vi "Fix_multi_header_bug.vi"(1 "Raw data File to Read":path) -> (0 "Raw data File to Read Out":path)   [LabVIEW 2018]
uses:
  Globals/Meas_global.vi
  Globals/Constants_global.vi
panel:
  out "character string":string
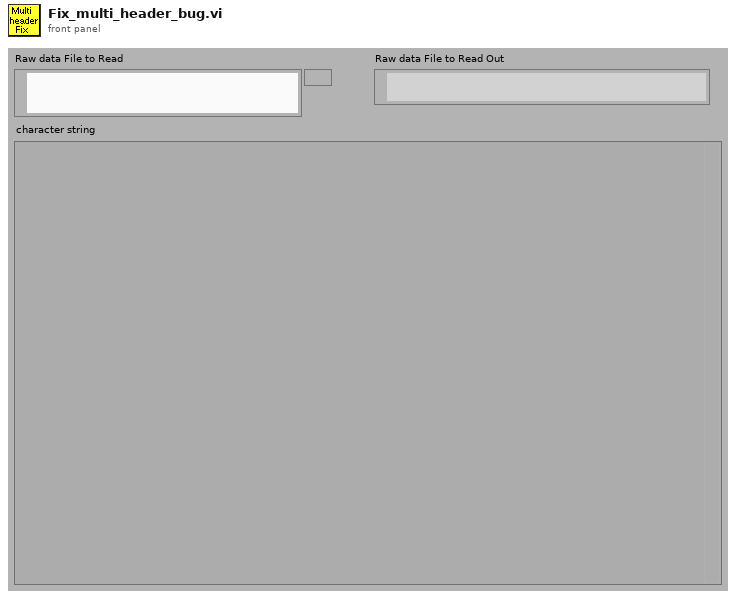
[diagram p1: front panel]
types:
  T1 = enum16{"read/write", "read-only", "write-only", "write-only (truncate)"}
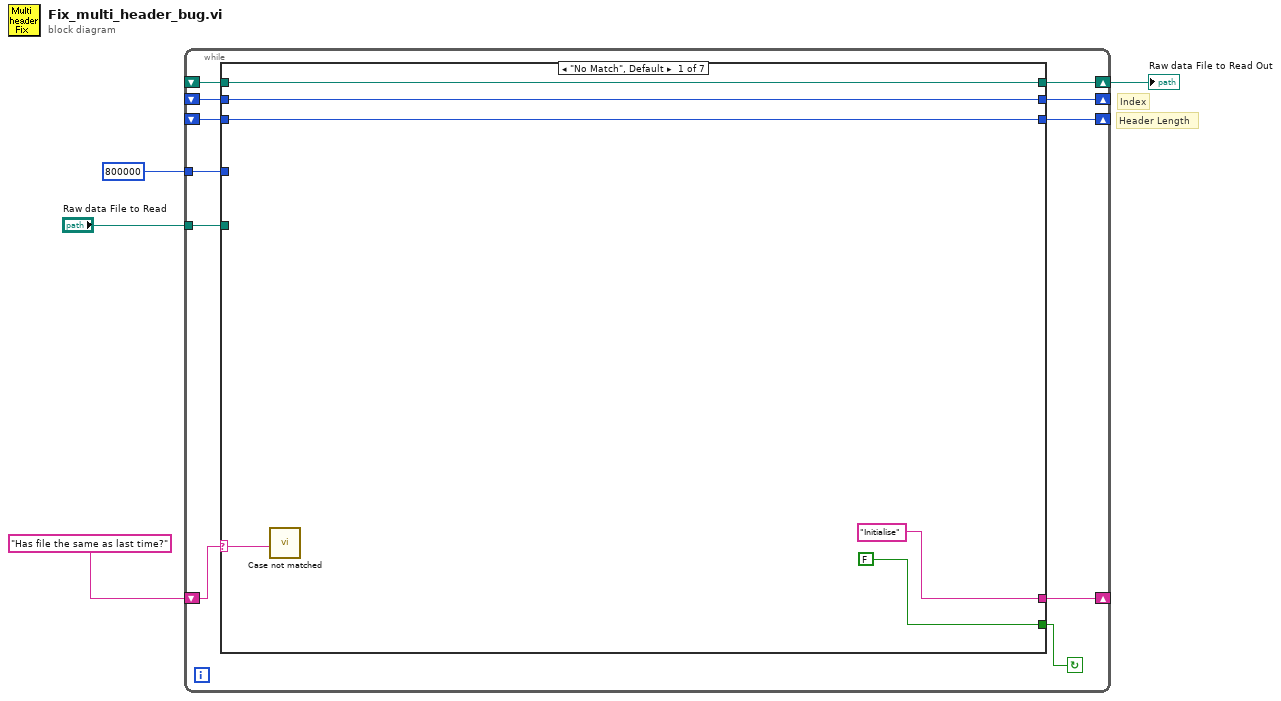
[diagram p0: block diagram]
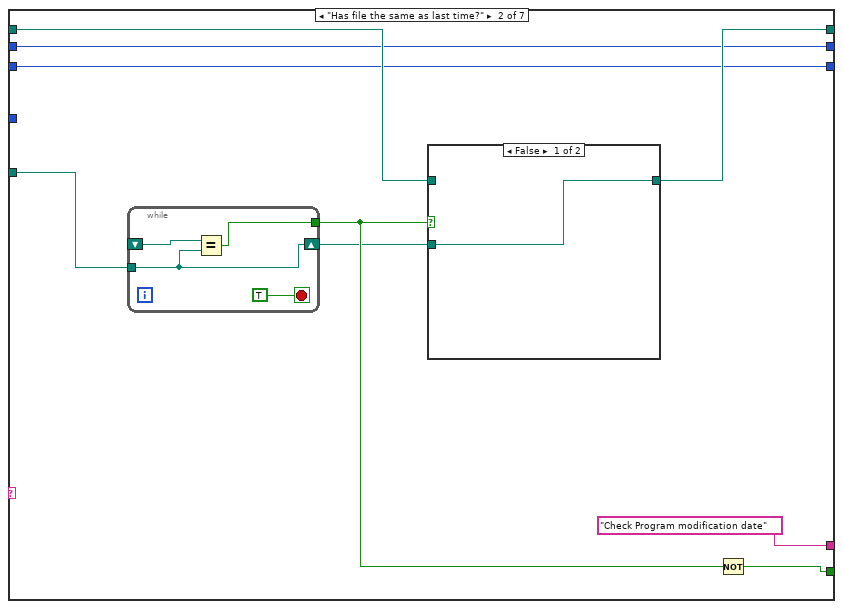
[diagram p2: hidden frame]
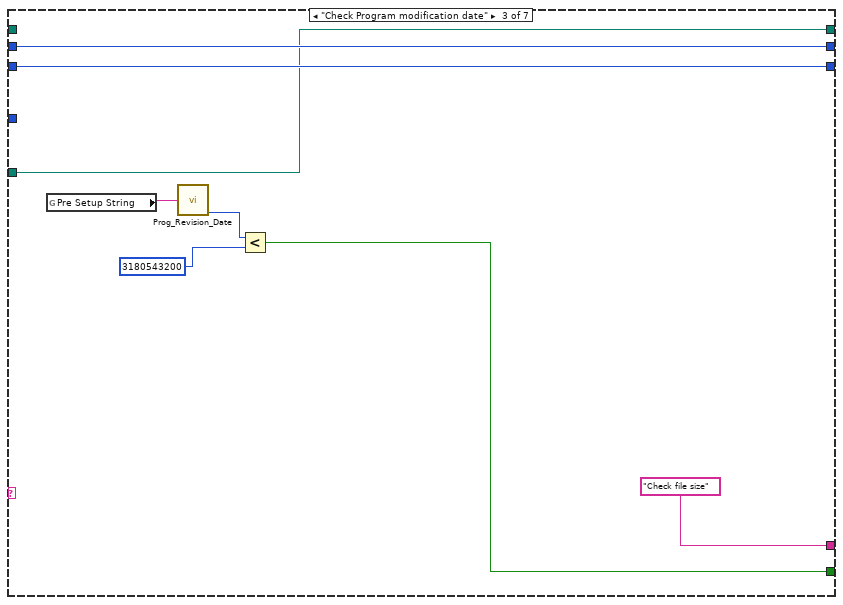
[diagram p4: hidden frame]
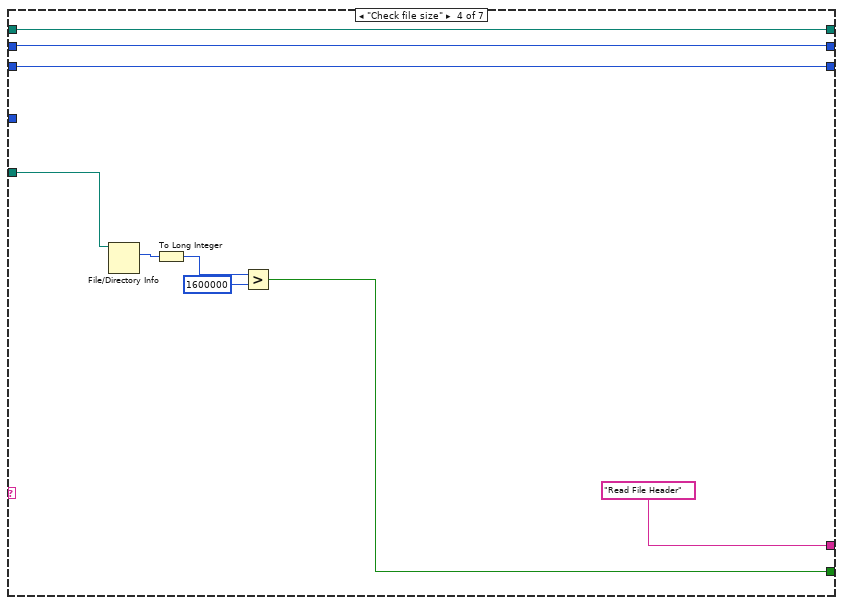
[diagram p5: hidden frame]
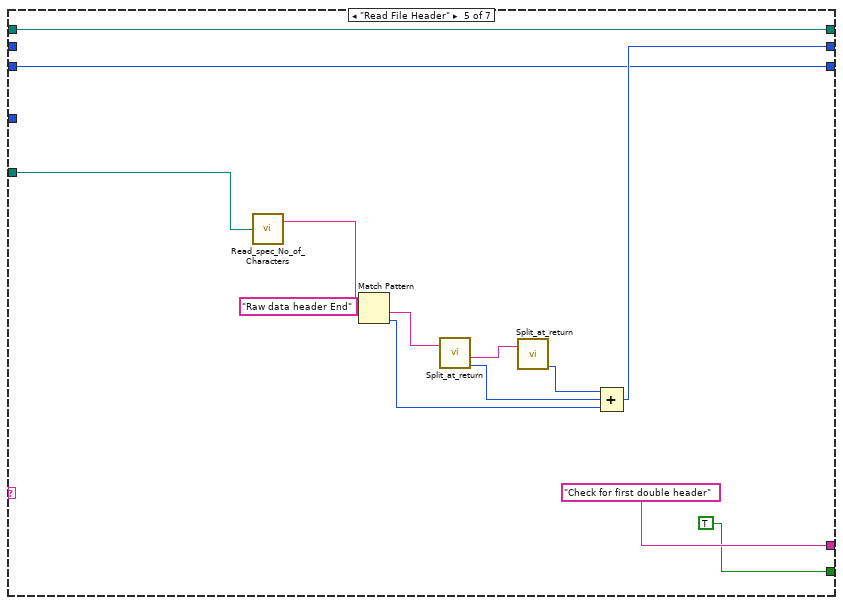
[diagram p6: hidden frame]
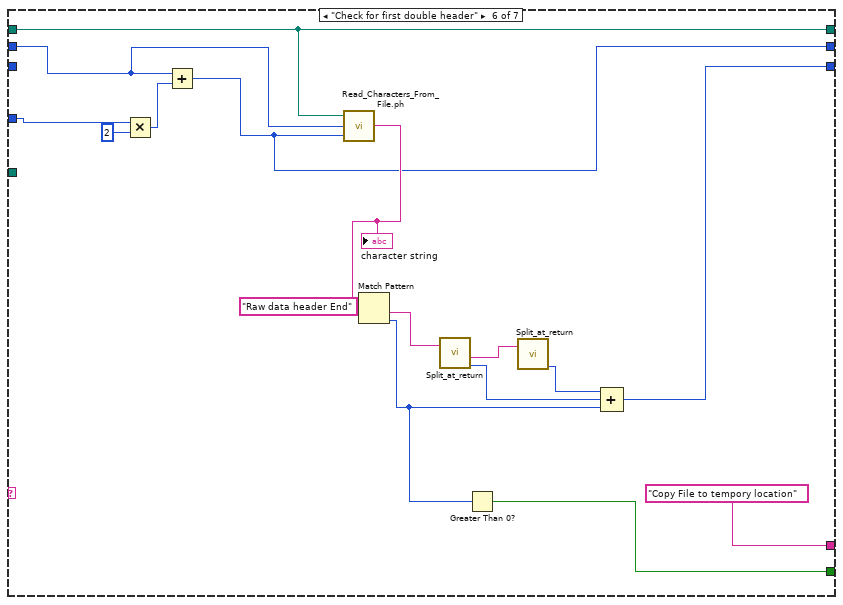
[diagram p7: hidden frame]
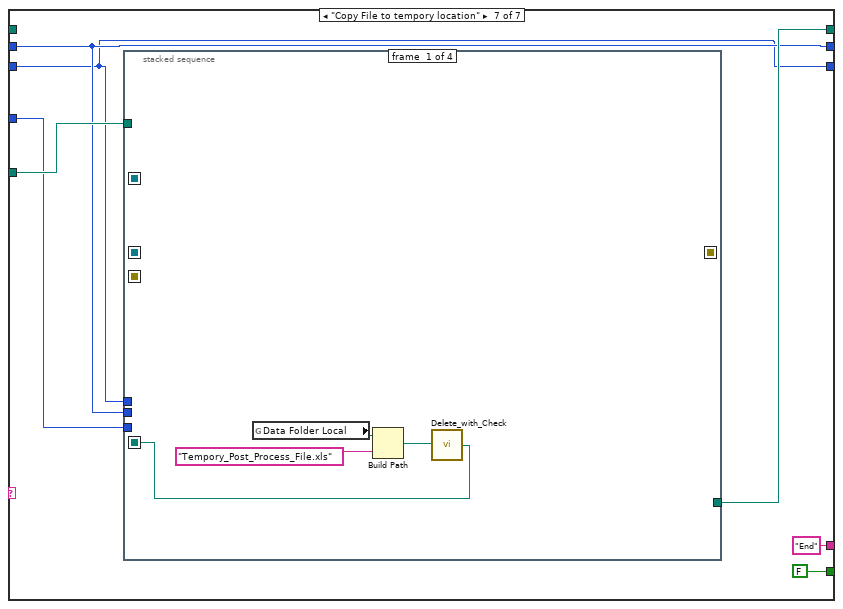
[diagram p8: hidden frame]
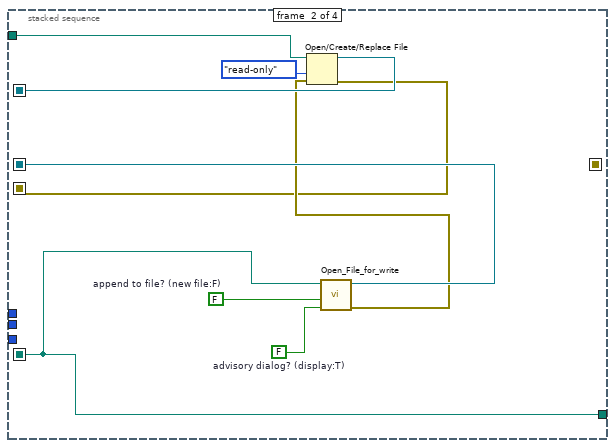
[diagram p9: hidden frame]
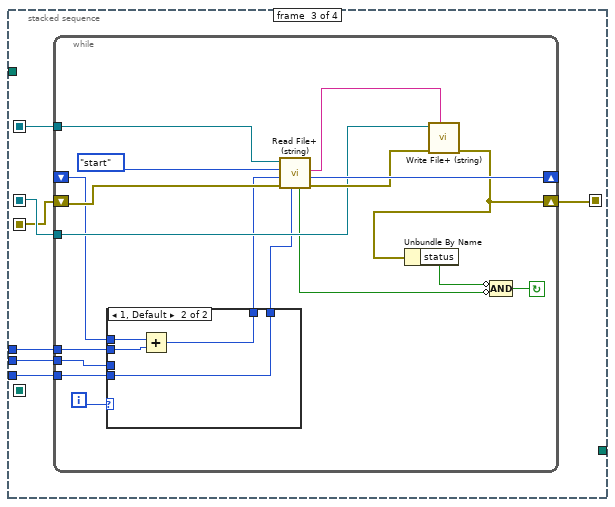
[diagram p10: hidden frame]
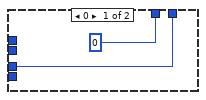
[diagram p11: hidden frame]
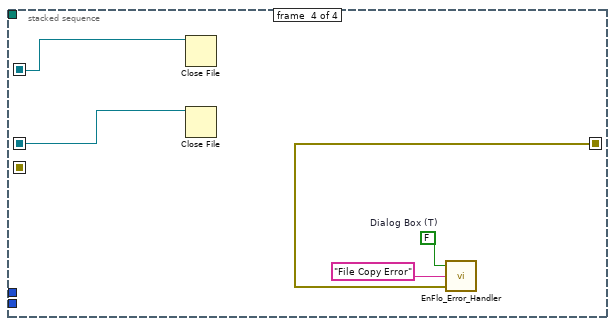
[diagram p12: hidden frame]
diagram:
  # "Header Length"
  # "Index"
  n1 = while {
    shift-left: "Has file the same as last time?" -> [w13]
    shift-right: [w14] -> _
    tunnel: "Raw data File to Read" -> [w12]
    shift-right: [w5] -> w2
    shift-left: _ -> [w11]
    shift-right: [w10] -> _
    shift-left: _ -> [w9]
    tunnel: 800000 -> [w8]
    shift-right: [w7] -> _
    shift-left: _ -> [w6]
    stop <- w15 continue-if-true
    n2 = case shown="\"No Match\", Default" w13 {
      selector: w13 -> [w16 _ _ _ _ _ _]
      tunnel: [FALSE w24 w43 w49 TRUE w69 FALSE] -> w15
      tunnel: ["Initialise" "Check Program modification date" "Check file size" "Read File Header" "Check for first double header" "Copy File to tempory location" "End"] -> w14
      tunnel: w12 -> [_ w30 w39 w52 w64 _ w89]
      tunnel: [w19 w29 w39 w46 w63 w73 w88] -> w5
      tunnel: w11 -> [w19 w28 _ w46 w63 w73 _]
      tunnel: [w18 w27 w41 w48 w55 w67 w84] -> w10
      tunnel: w9 -> [w18 w27 w41 w48 _ w71 w84]
      tunnel: w8 -> [_ _ _ _ _ w76 w87]
      tunnel: [w17 w26 w40 w47 w54 w68 w83] -> w7
      tunnel: w6 -> [w17 w26 w40 w47 w54 _ w83]
      frame "No Match", Default {
        n3 = call "Case not matched.vi"("Case Name not Matched"=w16) -> ()
      }
      frame "Has file the same as last time?" {
        n4 = while {
          shift-right: [w36] -> w22
          shift-left: _ -> [w35]
          tunnel: w30 -> [w36]
          tunnel: [w34] -> w25
          stop <- TRUE stop-if-true
          n5 = Equal?(x=w35, y=w36) -> (x = y?=w34:bool)
        }
        n6 = case shown="False" w25 {
          tunnel: [w31 w32] -> w29
          tunnel: w28 -> [_ w32]
          tunnel: w22 -> [w31 _]
          frame False {
          }
          frame True {
          }
        }
        n7 = Not(x=w25) -> (.not. x?=w24:bool)
      }
      frame "Check Program modification date" {
        n8 = global read "Meas_global.vi" "Pre Setup String"() -> (w38:string)
        n9 = call "Prog_Revision_Date.vi"("Input string"=w38) -> ("Revision time (s)"=w37:u32)  [unwired: 4 out]
        n10 = Less?(x=w37, y=u32 3180543200 ("Prog's last revision date")) -> (x < y?=w43:bool)
      }
      frame "Check file size" {
        n11 = File/Directory Info(path=w52) -> (size=w45:i64)  [unwired: 1 in, 6 out]
        n12 = To Long Integer(number=w45) -> (32bit integer=w51:i32)
        n13 = Greater?(x=w51, y=1600000) -> (0:w49:bool)
      }
      frame "Read File Header" {
        n14 = call "Read_spec_No_of_Characters.vi"("Filename"=w64) -> ("character string"=w61:string)  [unwired: 1 out]
        n15 = Match Pattern(string=w61, regular expression="Raw data header End") -> (after substring=w59:string, offset past match=w57:i32)  [unwired: 3 out]
        n16 = call "Split_at_return.vi"("String"=w59) -> ("after substring"=w60:string, "offset past match"=w56:i32)  [unwired: 1 in, 2 out]
        n17 = call "Split_at_return.vi"("String"=w60) -> ("offset past match"=w58:i32)  [unwired: 1 in, 3 out]
        n18 = Compound Arithmetic op=ADD(w58, w56, w57) -> (w55:i32)
      }
      frame "Check for first double header" {
        n19 = Multiply(x=w76, y=2) -> (x*y=w75:i32)
        n20 = Add(x=w71, y=w75) -> (x+y=w67:i32)
        n21 = call "Read_Characters_From_File.ph.vi"("file path (dialog if empty)"=w73, "number of characters (all:-1)"=w71, "start of read offset (chars.: 0)"=w67) -> ("character string"=w72:string)  [unwired: 6 out]
        "character string" <- w72
        n22 = Match Pattern(string=w72, regular expression="Raw data header End") -> (after substring=w79:string, offset past match=w70:i32)  [unwired: 3 out]
        n23 = call "Split_at_return.vi"("String"=w79) -> ("after substring"=w80:string, "offset past match"=w77:i32)  [unwired: 1 in, 2 out]
        n24 = Greater Than 0?(x=w70) -> (x > 0?=w69:bool)
        n25 = call "Split_at_return.vi"("String"=w80) -> ("offset past match"=w78:i32)  [unwired: 1 in, 3 out]
        n26 = Compound Arithmetic op=ADD(w78, w77, w70) -> (w68:i32)
      }
      frame "Copy File to tempory location" {
        n27 = stacked-sequence {
          seq-local: [_ w99 _ _] -> [_ _ w109 w138]
          seq-local: [_ w101 _ _] -> [_ _ w108 w137]
          seq-local: [_ w97 _ _] -> [_ _ w107 _]
          seq-local: [_ _ w106 _] -> [_ _ _ w135]
          seq-local: [w90 _ _ _] -> [_ w94 _ _]
          tunnel: w89 -> [_ w95 _ _]
          tunnel: [_ w94 _ _] -> w88
          tunnel: w84 -> [_ _ w105 _]
          tunnel: w83 -> [_ _ w104 _]
          tunnel: w87 -> [_ _ w103 _]
          frame #0 {
            n28 = global read "Constants_global.vi" "Data Folder Local"() -> (w92:path)
            n29 = Build Path(base path=w92, name or relative path="Tempory_Post_Process_File.xls") -> (appended path=w91:path)
            n30 = call "Delete_with_Check.vi"("FilePath"=w91) -> ("Deleted Filepath"=w90:path)
          }
          frame #1 {
            w96 = FALSE  # advisory dialog? (display:T)
            w102 = FALSE  # append to file? (new file:F)
            n31 = call "Open_File_for_write.vi"("advisory dialog? (display:T)"=w96, "append to file? (new file:F)"=w102, "file path"=w94) -> ("error out"=w98:errorcluster, "refnum"=w101:refnum<file>)  [unwired: 7 out]
            n32 = Open/Create/Replace File(file path (use dialog)=w95, error in=w98, access (0:read/write)=T1."read-only" ("open mode (0)")) -> (refnum out=w99:refnum<file>, error out=w97:errorcluster)  [unwired: 4 out]
          }
          frame #2 {
            n33 = while {
              shift-left: w107 -> [w121]
              shift-right: [w120] -> w106
              tunnel: w108 -> [w123]
              shift-left: _ -> [w112]
              shift-right: [w125] -> _
              tunnel: w109 -> [w126]
              tunnel: w105 -> [w114]
              tunnel: w104 -> [w111]
              tunnel: w103 -> [w110]
              i -> [w116]
              stop <- w117 continue-if-true
              n34 = case shown="1, Default" w116 {
                tunnel: [w129 w130] -> w115
                tunnel: w114 -> [w129 _]
                tunnel: [0 ("mark after read (bytes)") w131] -> w113
                tunnel: w112 -> [_ w133]
                tunnel: w111 -> [_ w132]
                tunnel: w110 -> [_ w130]
                frame 0 {
                }
                frame 1, Default {
                  n35 = Add(x=w133, y=w132) -> (x+y=w131:i32)
                }
              }
              n36 = call <vilib>:"Read File+ (string).vi"("count"=w115, "error in (no error)"=w121, "pos offset (bytes:0)"=w113, "pos mode (rel. to current:2)"=enum16{"start", "end", "current"}."start", "refnum"=w126) -> ("error out"=w124:errorcluster, "mark after read (bytes)"=w125:i32, "string"=w122:string, "EOF?"=w118:bool)  [unwired: 3 out]
              n37 = call <vilib>:"Write File+ (string).vi"("string"=w122, "error in (no error)"=w124, "refnum"=w123) -> ("error out"=w120:errorcluster)  [unwired: 2 in, 4 out]
              n38 = Unbundle By Name(w120) -> ("status"=w119:bool)
              n39 = Compound Arithmetic op=AND(invert w119, invert w118) -> (w117:bool)
            }
          }
          frame #3 {
            w136 = FALSE  # Dialog Box (T)
            n40 = Close File(refnum=w138) -> ()  [unwired: 1 in, 2 out]
            n41 = Close File(refnum=w137) -> ()  [unwired: 1 in, 2 out]
            n42 = call "EnFlo_Error_Handler.vi"("error in (no error)"=w135, "Error Type"="File Copy Error", "Dialog Box (T)"=w136) -> ()  [unwired: 3 out]
          }
        }
      }
    }
  }
  "Raw data File to Read Out" <- w2
